vi "Database Command Set Stored Procedure Text.vi"(7 "Prepare?":bool, 8 "error in (no error)":errorcluster caption="错误输入（无错误）", 10 "CommandText":string, 11 "Database Command 输入":refnum<class "Database Command.lvclass"> caption="DNL_LabVIEW Object in") -> (0 "error out":errorcluster caption="错误输出", 3 "Database Command 输出":refnum<class "Database Command.lvclass"> caption="DNL_LabVIEW Object out")   [LabVIEW 2011, in "Database Command.lvclass"]
uses:
  Database Command.lvclass
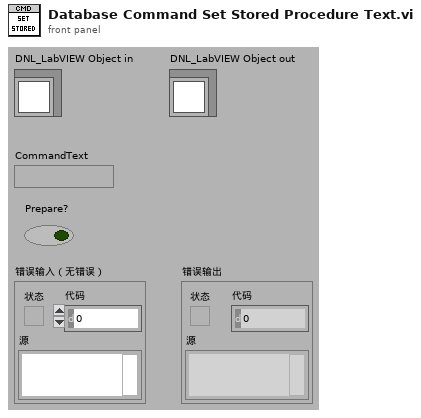
[diagram p1: front panel]
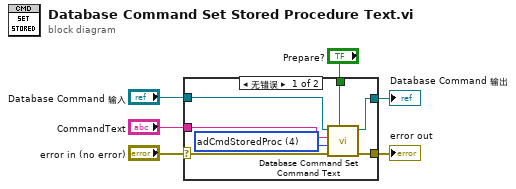
[diagram p0: block diagram]
diagram:
  n1 = case shown="无错误" "error in (no error)" {
    selector: "error in (no error)" -> [w8 w15]
    tunnel: [w7 w15] -> w5
    tunnel: [w12 w14] -> w3
    tunnel: "Database Command 输入" -> [w13 w14]
    tunnel: "Prepare?" -> [w11 _]
    tunnel: "CommandText" -> [w10 _]
    frame No Error {
      w9 = 4 items=["adCmdUnspecified"=-1, "adCmdUnknown"=8, "adCmdText"=1, "adCmdTable"=2, "adCmdStoredProc"=4, "adCmdFile"=256, "adCmdTableDirect"=512] ("CommandType")
      n2 = call "Database Command Set Command Text.vi"("Prepared"=w11, "error in (no error)"=w8, "CommandType"=w9, "CommandText"=w10, "Database Command 输入"=w13) -> ("error out"=w7:errorcluster, "Database Command 输出"=w12:refnum<class "Database Command.lvclass">)  [unwired: 5 in]
    }
    frame Error {
    }
  }
  "error out" <- w5
  "Database Command 输出" <- w3
